vi "Save Settings.vi"(8 "error in (no error)":errorcluster {"code" format="Error %.0f"}, 11 "VIDoc Settings In":refnum<class "VIDoc Settings.lvclass">) -> (0 "error out":errorcluster {"code" format="Error %.0f"}, 3 "VIDoc Settings Out":refnum<class "VIDoc Settings.lvclass">)   [LabVIEW 2023, in "VIDoc Settings.lvclass"]
uses:
  VIDoc Settings.lvclass
  VIDoc Settings.lvclass/VIDoc Settings.ctl
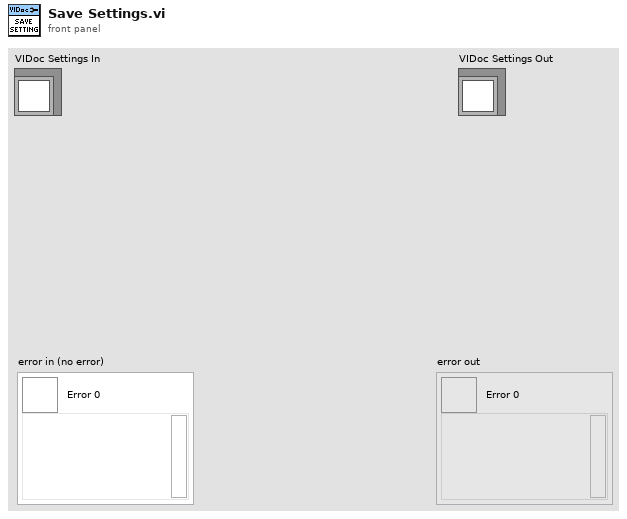
[diagram p1: front panel]
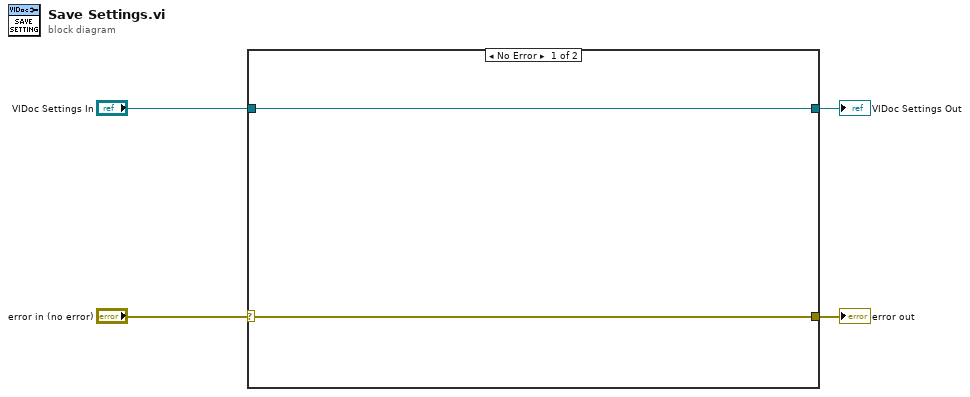
[diagram p0: block diagram]
diagram:
  n1 = case shown="No Error" "error in (no error)" {
    selector: "error in (no error)" -> [w5 w8]
    tunnel: [w5 w8] -> w3
    tunnel: [w6 w7] -> w1
    tunnel: "VIDoc Settings In" -> [w6 w7]
    frame No Error {
    }
    frame Error {
    }
  }
  "error out" <- w3
  "VIDoc Settings Out" <- w1
